vi "Queue FGV.vi"(8 "error in (no error)":errorcluster, 10 "Action":T1=enum."Release", 11 "Queue In":refnum<queue>) -> (0 "error out":errorcluster, 3 "Queue Out":refnum<queue>)   [LabVIEW 2014, in "Control Module.lvlib"]
uses:
  Control Module.lvlib
  Queue FGV.ctl
  Message.ctl
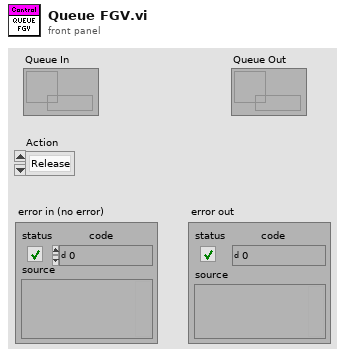
[diagram p1: front panel]
types:
  T1 = typedef "Control Module.lvlib/Queue FGV.ctl" = enum16{"Set", "Get", "Release"}
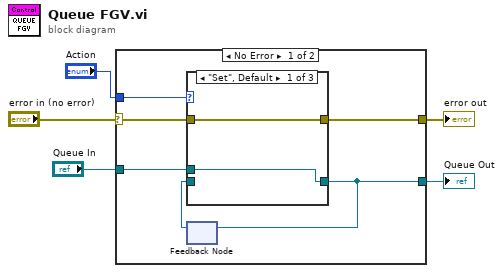
[diagram p0: block diagram]
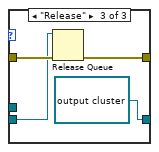
[diagram p3: hidden frame]
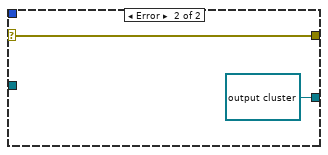
[diagram p4: hidden frame]
diagram:
  n1 = case shown="No Error" "error in (no error)" {
    selector: "error in (no error)" -> [w10 w21]
    tunnel: [w9 w21] -> w5
    tunnel: "Action" -> [w11 _]
    tunnel: [w7 refnum<queue> refnum ("queue out")] -> w1
    tunnel: "Queue In" -> [w6 _]
    frame No Error {
      n2 = feedback #1() -> (w8:refnum<queue>)  [unwired: 1 in]
      n3 = case shown="\"Set\", Default" w11 {
        tunnel: w10 -> [w13 w15 w19]
        tunnel: [w13 w15 w18] -> w9
        tunnel: [w12 w14 refnum<queue> refnum ("queue out")] -> w7
        tunnel: w8 -> [_ w14 w16]
        tunnel: w6 -> [w12 _ _]
        frame "Set", Default {
        }
        frame "Get" {
        }
        frame "Release" {
          n4 = Release Queue(queue=w16, error in (no error)=w19) -> (error out=w18:errorcluster)  [unwired: 1 in, 2 out]
        }
      }
      n5 = feedback-in #1(w7) -> ()
    }
    frame Error {
    }
  }
  "error out" <- w5
  "Queue Out" <- w1
